vi "Lognormal CDF.vi"(9 "c":dbl=3.0, 10 "b":dbl=2.0, 11 "x":dbl=1.0) -> (0 "error":i32, 3 "cdf(x)":dbl=0.40863834423098205)   [LabVIEW 2014, in "NI_Gmath.lvlib"]
doc: "Computes the continuous cumulative distribution function (CDF), or the probability that the random variate X, where X describes the selected distribution type, has a value less than or equal to <B>x</B>. You must manually select the polymorphic instance to use."
uses:
  NI_Gmath.lvlib
  st_error_code.ctl
panel:
  # "Lognormal CDF"
  # "median (scale)"
  # "standard dev (shape)"
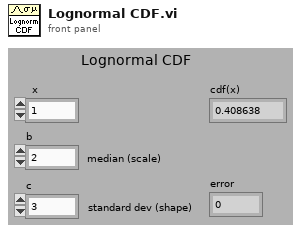
[diagram p1: front panel]
types:
  T1 = typedef "NI_Gmath.lvlib/st_error_code.ctl" = i32
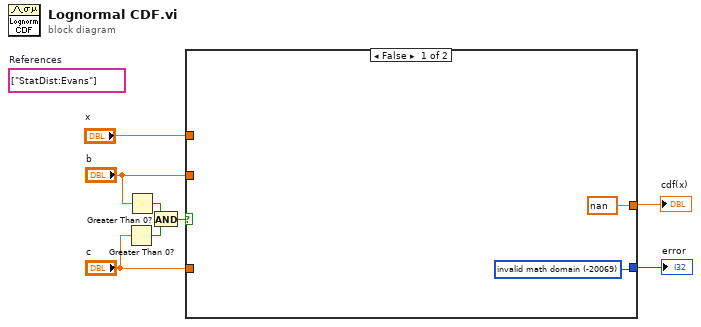
[diagram p0: block diagram]
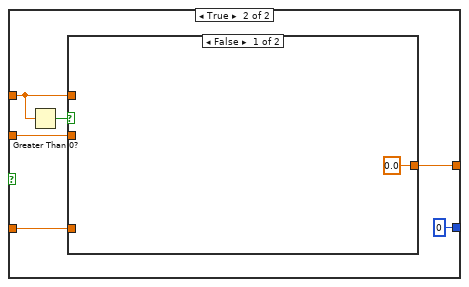
[diagram p2: hidden frame]
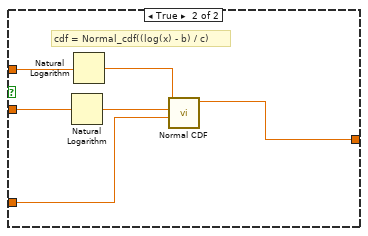
[diagram p3: hidden frame]
diagram:
  (unwired) string[] ["StatDist:Evans"]  # References
  n1 = Greater Than 0?(x="c") -> (x > 0?=w6:bool)
  n2 = Greater Than 0?(x="b") -> (x > 0?=w7:bool)
  n3 = And(x=w7, y=w6) -> (x .and. y?=w8:bool)
  n4 = case shown="False" w8 {
    tunnel: "c" -> [_ w13]
    tunnel: [w9 0 ("invalid math domain")] -> w1
    tunnel: [nan w14] -> w2
    tunnel: "x" -> [_ w11]
    tunnel: "b" -> [_ w15]
    frame False {
      w9 = T1 -20069 items=["invalid math domain"=-20069, "Fourier interpolation size m >= n"=-20070, "empty array"=-20003] ("stat interp error code")
    }
    frame True {
      n5 = Greater Than 0?(x=w11) -> (x > 0?=w12:bool)
      n6 = case shown="False" w12 {
        tunnel: w15 -> [_ w21]
        tunnel: [0.0 w19] -> w14
        tunnel: w11 -> [_ w23]
        tunnel: w13 -> [_ w20]
        frame False {
        }
        frame True {
          # "cdf = Normal_cdf((log(x) - b) / c)"
          n7 = Natural Logarithm(1:w21) -> (0:w18:dbl)
          n8 = Natural Logarithm(1:w23) -> (0:w22:dbl)
          n9 = call "Normal CDF.vi"("std"=w20, "mean"=w18, "x"=w22) -> ("cdf(x)"=w19:dbl)  [unwired: 7 in, 1 out]
        }
      }
    }
  }
  "cdf(x)" <- w2
  "error" <- w1
